vi "FunctionClass.vi"(8 "error in (no error)":errorcluster, 10 "FunctionClass":variant, 11 "ModuleID":i32) -> (0 "error out":errorcluster)   [LabVIEW 2018, in "AnalysisModule.lvlib"]
uses:
  AnalysisModule.lvlib
  clEventType.ctl
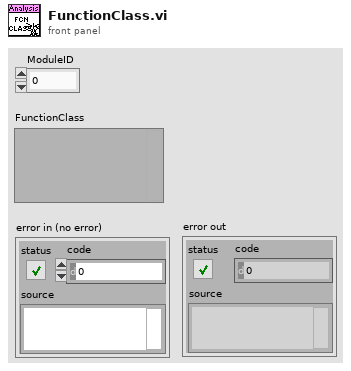
[diagram p1: front panel]
types:
  T1 = typedef "AnalysisModule.lvlib/clEventType.ctl" = cluster{"ModuleID":i32, "Data":variant}
  T2 = typedef "AnalysisModule.lvlib/clBroadcastEvents.ctl" = cluster{"DidInit":refnum<user-event>, "StatusUpdate":refnum<user-event>, "ErrorReport":refnum<user-event>, "DidStop":refnum<user-event>, "PathToINI":refnum<user-event>, "Config":refnum<user-event>, "ResultReport":refnum<user-event>, "FunctionClass":refnum<user-event>}
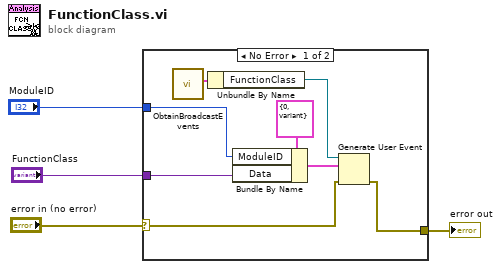
[diagram p0: block diagram]
diagram:
  n1 = case shown="No Error" "error in (no error)" {
    selector: "error in (no error)" -> [w6 w13]
    tunnel: "ModuleID" -> [w11 _]
    tunnel: [w5 w13] -> w3
    tunnel: "FunctionClass" -> [w7 _]
    frame No Error {
      n2 = call "ObtainBroadcastEvents.vi"() -> ("clBroadcastEvents"=w10:T2)  [unwired: 10 in, 1 out]
      n3 = Unbundle By Name(w10) -> ("FunctionClass"=w8:refnum<user-event>)
      n4 = Bundle By Name(cluster=T1 {"ModuleID"=0, "Data"=variant} ("clEventType"), "ModuleID"=w11, "Data"=w7) -> (w9:T1)
      n5 = Generate User Event(user event=w8, event data cluster=w9, error in=w6) -> (error out=w5:errorcluster)  [unwired: 1 in, 1 out]
    }
    frame Error {
    }
  }
  "error out" <- w3
